vi "log analysis_gps.vi"() -> ()   [LabVIEW 2019] (continued)
31T\",12,5,5,3,04,00,20,03*fd84ab6f\n\tsystem status\tnormal 2 27.900000 0 0\trobot status\t165.672494\t122.157041\t7.863900\t0.259103\t-0.236619\t173.916290\t0.293000\t0.003000\n\t\n15:43:45.0\tlog_raw\tgps_raw\t#DUALANTENNAHEADINGA,USB3,0,47.0,FINESTEERING,2107,283443.000,02000000,d426,15824;INSUFFICIENT_OBS,NONE,-1.000000000,0.000000000,0.000000000,0.0,0.000000000,0.000000000,\"631T\",12,4,4,3,04,00,20,03*cb2f73ac\n\tsystem status\tnormal 2 27.900000 0 0\trobot status\t165.523586\t122.191427\t7.865700\t0.210877\t-0.293700\t173.825289\t0.305000\t0.013000\n\t\n15:43:45.5\tlog_raw\tgps_raw\t#DUALANTENNAHEADINGA,USB3,0,50.0,FINESTEERING,2107,283443.500,02000000,d426,15824;SOL_COMPUTED,L1_FLOAT,-1.000000000,232.711517334,45.470851898,0.0,33.751167297,39.018550873,\"631T\",12,5,5,3,04,00,20,03*51b2f499\n\tsystem status\tnormal 2 27.900000 0 0\trobot status\t165.380662\t122.222844\t7.868200\t0.351026\t-0.300668\t173.767121\t0.301000\t0.006000\n\t\n15:43:46.0\tlog_raw\tgps_raw\t#DUALANTENNAHEADINGA,USB3,0,50.0,FINESTEERING,2107,283444.000,02000000,d426,15824;INSUFFICIENT_OBS,NONE,-1.000000000,0.000000000,0.000000000,0.0,0.000000000,0.000000000,\"631T\",13,4,4,3,04,00,20,03*f1c4efa0\n\tsystem status\tnormal 2 27.900000 0 0\trobot status\t165.233504\t122.257140\t7.870500\t0.509598\t-0.309448\t173.742024\t0.303000\t0.009000\n\t\n15:43:46.5\tlog_raw\tgps_raw\t#DUALANTENNAHEADINGA,USB3,0,48.0,FINESTEERING,2107,283444.500,02000000,d426,15824;INSUFFICIENT_OBS,NONE,-1.000000000,0.000000000,0.000000000,0.0,0.000000000,0.000000000,\"631T\",13,4,4,3,04,00,20,03*63cc647c\n\tsystem status\tnormal 2 27.900000 0 0\trobot status\t165.100809\t122.287890\t7.873300\t0.523177\t-0.494729\t173.684348\t0.299000\t-0.035000\n\t\n15:43:47.0\tlog_raw\tgps_raw\t#DUALANTENNAHEADINGA,USB3,0,48.0,FINESTEERING,2107,283445.000,02000000,d426,15824;INSUFFICIENT_OBS,NONE,-1.000000000,0.000000000,0.000000000,0.0,0.000000000,0.000000000,\"631T\",13,4,4,3,04,00,20,03*d90771fc\n\tsystem status\tnormal 2 27.900000 0 0\trobot status\t164.960140\t122.320641\t7.876000\t0.439094\t-0.529708\t173.639540\t0.358000\t-0.023000\n\t\n15:43:47.5\tlog_raw\tgps_raw\t#INSPVAXA,USB3,0,43.5,FINESTEERING,2107,283445.500,02000000,471d,15824;INS_ALIGNMENT_COMPLETE,INS_RTKFIXED,37.37123259759,126.72269590770,7.8782,22.3000,0.0945,-0.3330,-0.0049,0.334033623,-0.428396374,276.205094266,0.4384,0.2941,0.5693,0.1131,0.0924,0.0780,0.0965,0.1014,4.9958,0f000001,0*eef193fc\n\tsystem status\tnormal 2 27.900000 0 0\trobot status\t164.826847\t122.347921\t7.878200\t0.334034\t-0.428396\t173.794906\t0.303000\t0.000000\n\t\n15:43:48.0\tlog_raw\tgps_raw\t#DUALANTENNAHEADINGA,USB3,0,43.5,FINESTEERING,2107,283446.000,02000000,d426,15824;INSUFFICIENT_OBS,NONE,-1.000000000,0.000000000,0.000000000,0.0,0.000000000,0.000000000,\"631T\",12,4,4,3,04,00,20,03*d5fed84d\n\tsystem status\tnormal 2 27.800000 0 0\trobot status\t164.679034\t122.378754\t7.879600\t0.256661\t-0.601518\t173.977970\t0.256000\t0.060000\n\t\n15:43:48.5\tlog_raw\tgps_raw\t#INSPVAXA,USB3,0,50.0,FINESTEERING,2107,283446.500,02000000,471d,15824;INS_ALIGNMENT_COMPLETE,INS_RTKFIXED,37.37123311226,126.72269261048,7.8801,22.3000,0.1011,-0.2963,-0.0025,0.185692893,-0.737548130,275.721839304,0.4376,0.2941,0.5694,0.1127,0.0923,0.0781,0.0965,0.1014,4.9971,0f000001,0*33922ff8\n\tsystem status\tnormal 2 27.800000 0 0\trobot status\t164.534785\t122.405047\t7.880100\t0.185693\t-0.737548\t174.278161\t0.270000\t0.050000\n\t\n15:43:49.0\tlog_raw\tgps_raw\t#DUALANTENNAHEADINGA,USB3,0,50.0,FINESTEERING,2107,283447.000,02000000,d426,15824;INSUFFICIENT_OBS,NONE,-1.000000000,0.000000000,0.000000000,0.0,0.000000000,0.000000000,\"631T\",11,4,4,3,04,00,20,03*3318e43a\n\tsystem status\tnormal 2 27.800000 0 0\trobot status\t164.391452\t122.433038\t7.880200\t0.201760\t-0.895547\t174.637577\t0.423000\t-0.172000\n\t\n15:43:49.5\tlog_raw\tgps_raw\t\tsystem status\tnormal 2 27.800000 0 0\trobot status\t164.251464\t122.459981\t7.881400\t0.307007\t-0.942643\t175.000438\t0.380000\t-0.105000\n\t\n15:43:50.0\tlog_raw\tgps_raw\t\tsystem status\tnormal 2 27.800000 0 0\trobot status\t164.109642\t122.487191\t7.882000\t0.246007\t-0.944004\t175.404925\t0.310000\t0.000000\n\t\n15:43:50.5\tlog_raw\tgps_raw\t#DUALANTENNAHEADINGA,USB3,0,51.5,FINESTEERING,2107,283448.500,02000000,d426,15824;INSUFFICIENT_OBS,NONE,-1.000000000,0.000000000,0.000000000,0.0,0.000000000,0.000000000,\"631T\",14,4,4,3,04,00,20,03*e9e47ab5\n\tsystem status\tnormal 2 27.800000 0 0\trobot status\t163.966863\t122.507000\t7.881200\t0.146187\t-0.918607\t175.866962\t0.302000\t0.000000\n\t\n15:43:51.0\tlog_raw\tgps_raw\t#DUALANTENNAHEADINGA,USB3,0,51.5,FINESTEERING,2107,283449.000,02000000,d426,15824;INSUFFICIENT_OBS,NONE,-1.000000000,0.000000000,0.000000000,0.0,0.000000000,0.000000000,\"631T\",12,4,4,3,04,00,20,03*cef36426\n\tsystem status\tnormal 2 27.800000 0 0\trobot status\t163.825609\t122.528899\t7.879700\t0.116711\t-0.792490\t176.146644\t0.187000\t0.125000\n\t\n15:43:51.5\tlog_raw\tgps_raw\t\tsystem status\tnormal 2 27.800000 0 0\trobot status\t163.693916\t122.547630\t7.877800\t0.151929\t-0.650163\t176.408867\t0.313000\t0.002000\n\t\n15:43:52.0\tlog_raw\tgps_raw\t#DUALANTENNAHEADINGA,USB3,0,49.0,FINESTEERING,2107,283450.000,02000000,d426,15824;INSUFFICIENT_OBS,NONE,-1.000000000,0.000000000,0.000000000,0.0,0.000000000,0.000000000,\"631T\",14,4,4,3,04,00,20,03*09d68f9b\n\tsystem status\tnormal 2 27.800000 0 0\trobot status\t163.555418\t122.571158\t7.876300\t0.483832\t-0.633082\t176.720348\t0.260000\t0.076000\n\t\n15:43:52.5\tlog_raw\tgps_raw\t#DUALANTENNAHEADINGA,USB3,0,49.0,FINESTEERING,2107,283450.500,02000000,d426,15824;INSUFFICIENT_OBS,NONE,-1.000000000,0.000000000,0.000000000,0.0,0.000000000,0.000000000,\"631T\",12,4,4,3,04,00,20,03*431995d1\n\tsystem status\tnormal 2 27.800000 0 0\trobot status\t163.413955\t122.592581\t7.875300\t0.523841\t-0.742821\t176.868735\t0.267000\t0.059000\n\t\n15:43:53.0\tlog_raw\tgps_raw\t#DUALANTENNAHEADINGA,USB3,0,49.0,FINESTEERING,2107,283451.000,02000000,d426,15824;INSUFFICIENT_OBS,NONE,-1.000000000,0.000000000,0.000000000,0.0,0.000000000,0.000000000,\"631T\",12,4,4,3,04,00,20,03*f9d28051\n\tsystem status\tnormal 2 27.900000 0 0\trobot status\t163.273523\t122.615568\t7.873300\t0.453873\t-0.748594\t176.979246\t0.320000\t-0.040000\n\t\n15:43:53.5\tlog_raw\tgps_raw\t#DUALANTENNAHEADINGA,USB3,0,44.5,FINESTEERING,2107,283451.500,02000000,d426,15824;INSUFFICIENT_OBS,NONE,-1.000000000,0.000000000,0.000000000,0.0,0.000000000,0.000000000,\"631T\",14,4,4,3,04,00,20,03*5c854f00\n\tsystem status\tnormal 2 27.900000 0 0\trobot status\t163.130518\t122.634911\t7.871300\t0.469672\t-0.900314\t177.008308\t0.303000\t-0.013000\n\t\n15:43:54.0\tlog_raw\tgps_raw\t#DUALANTENNAHEADINGA,USB3,0,44.5,FINESTEERING,2107,283452.000,02000000,d426,15824;INSUFFICIENT_OBS,NONE,-1.000000000,0.000000000,0.000000000,0.0,0.000000000,0.000000000,\"631T\",14,4,4,3,04,00,20,03*3dfe5332\n\tsystem status\tnormal 2 27.900000 0 0\trobot status\t162.988413\t122.656985\t7.869200\t0.628422\t-0.827167\t177.062583\t0.358000\t-0.086000\n\t\n15:43:54.5\tlog_raw\tgps_raw\t#DUALANTENNAHEADINGA,USB3,0,49.0,FINESTEERING,2107,283452.500,02000000,d426,15824;INSUFFICIENT_OBS,NONE,-1.000000000,0.000000000,0.000000000,0.0,0.000000000,0.000000000,\"631T\",12,4,4,3,04,00,20,03*98a99c63\n\tsystem status\tnormal 2 27.900000 0 0\trobot status\t162.847082\t122.675336\t7.867000\t0.701223\t-0.805865\t177.020983\t0.308000\t-0.011000\n\t\n15:43:55.0\tlog_raw\tgps_raw\t#DUALANTENNAHEADINGA,USB3,0,49.0,FINESTEERING,2107,283453.000,02000000,d426,15824;INSUFFICIENT_OBS,NONE,-1.000000000,0.000000000,0.000000000,0.0,0.000000000,0.000000000,\"631T\",10,4,4,3,04,00,20,03*56d68f12\n\tsystem status\tnormal 2 27.900000 0 0\trobot status\t162.707913\t122.695365\t7.863400\t0.653811\t-0.817944\t176.906378\t0.285000\t-0.006000\n\t\n15:43:55.5\tlog_raw\tgps_raw\t#DUALANTENNAHEADINGA,USB3,0,50.0,FINESTEERING,2107,283453.500,02000000,d426,15824;INSUFFICIENT_OBS,NONE,-1.000000000,0.000000000,0.000000000,0.0,0.000000000,0.000000000,\"631T\",9,4,4,3,04,00,20,02*71c65a10\n\tsystem status\tnormal 2 27.900000 0 0\trobot status\t162.567512\t122.713036\t7.859600\t0.640293\t-0.840166\t176.803743\t0.287000\t-0.006000\n\t\n15:43:56.0\tlog_raw\tgps_raw\t#DUALANTENNAHEADINGA,USB3,0,50.0,FINESTEERING,2107,283454.000,02000000,d426,15824;INSUFFICIENT_OBS,NONE,-1.000000000,0.000000000,0.000000000,0.0,0.000000000,0.000000000,\"631T\",10,4,4,3,04,00,20,03*adf0db7d\n\tsystem status\tnormal 2 27.900000 0 0\trobot status\t162.462286\t122.731023\t7.856300\t0.648331\t-0.862744\t176.715837\t0.257000\t0.003000\n\t\n15:43:56.5\tlog_raw\tgps_raw\t#DUALANTENNAHEADINGA,USB3,0,53.5,FINESTEERING,2107,283454.500,02000000,d426,15824;INSUFFICIENT_OBS,NONE,-1.000000000,0.000000000,0.000000000,0.0,0.000000000,0.000000000,\"631T\",10,4,4,3,04,00,20,03*83545704\n\tsystem status\tnormal 2 27.900000 0 0\trobot status\t162.317691\t122.747222\t7.853100\t0.502604\t-0.882304\t176.698904\t0.312000\t-0.030000\n\t\n15:43:57.0\tlog_raw\tgps_raw\t#DUALANTENNAHEADINGA,USB3,0,53.5,FINESTEERING,2107,283455.000,02000000,d426,15824;INSUFFICIENT_OBS,NONE,-1.000000000,0.000000000,0.000000000,0.0,0.000000000,0.000000000,\"631T\",10,4,4,3,04,00,20,03*399f4284\n\tsystem status\tnormal 2 27.900000 0 0\trobot status\t162.177621\t122.765962\t7.848800\t0.462674\t-0.849181\t176.541164\t0.296000\t-0.007000\n\t\n15:43:57.5\tlog_raw\tgps_raw\t#DUALANTENNAHEADINGA,USB3,0,53.0,FINESTEERING,2107,283455.500,02000000,d426,15824;INSUFFICIENT_OBS,NONE,-1.000000000,0.000000000,0.000000000,0.0,0.000000000,0.000000000,\"631T\",10,4,4,3,04,00,20,03*bbf6b511\n\tsystem status\tnormal 2 27.900000 0 0\trobot status\t162.042961\t122.783351\t7.845600\t0.471260\t-0.741428\t176.451320\t0.306000\t-0.003000\n\t\n15:43:58.0\tlog_raw\tgps_raw\t#DUALANTENNAHEADINGA,USB3,0,53.0,FINESTEERING,2107,283456.000,02000000,d426,15824;INSUFFICIENT_OBS,NONE,-1.000000000,0.000000000,0.000000000,0.0,0.000000000,0.000000000,\"631T\",10,4,4,3,04,00,20,03*da8da923\n\tsystem status\tnormal 2 27.900000 0 0\trobot status\t161.898614\t122.802999\t7.842000\t0.376839\t-0.675596\t176.320728\t0.295000\t-0.010000\n\t\n15:43:58.5\tlog_raw\tgps_raw\t#DUALANTENNAHEADINGA,USB3,0,50.5,FINESTEERING,2107,283456.500,02000000,d426,15824;INSUFFICIENT_OBS,NONE,-1.000000000,0.000000000,0.000000000,0.0,0.000000000,0.000000000,\"631T\",10,4,4,3,04,00,20,03*f429255a\n\tsystem status\tnormal 2 27.900000 0 0\trobot status\t161.764410\t122.820069\t7.837800\t0.218441\t-0.529178\t176.132166\t0.306000\t-0.016000\n\t\n15:43:59.0\tlog_raw\tgps_raw\t#DUALANTENNAHEADINGA,USB3,0,50.5,FINESTEERING,2107,283457.000,02000000,d426,15824;INSUFFICIENT_OBS,NONE,-1.000000000,0.000000000,0.000000000,0.0,0.000000000,0.000000000,\"631T\",11,4,4,3,04,00,20,03*9900b082\n\tsystem status\tnormal 2 27.900000 0 0\trobot status\t161.620308\t122.839916\t7.833300\t0.041782\t-0.506976\t175.942397\t0.298000\t-0.010000\n\t\n15:43:59.5\tlog_raw\tgps_raw\t#DUALANTENNAHEADINGA,USB3,0,52.0,FINESTEERING,2107,283457.500,02000000,d426,15824;INSUFFICIENT_OBS,NONE,-1.000000000,0.000000000,0.000000000,0.0,0.000000000,0.000000000,\"631T\",11,4,4,3,04,00,20,03*d3e0ea5f\n\tsystem status\tnormal 2 27.900000 0 0\trobot status\t161.478382\t122.859023\t7.830000\t0.076043\t-0.364293\t175.707938\t0.306000\t-0.023000\n\t\n15:44:00.0\tlog_raw\tgps_raw\t#DUALANTENNAHEADINGA,USB3,0,52.0,FINESTEERING,2107,283458.000,02000000,d426,15824;INSUFFICIENT_OBS,NONE,-1.000000000,0.000000000,0.000000000,0.0,0.000000000,0.000000000,\"631T\",12,4,4,3,04,00,20,02*d2f97f3d\n\tsystem status\tnormal 2 27.900000 0 0\trobot status\t161.335080\t122.881838\t7.825800\t0.229097\t-0.118774\t175.500608\t0.291000\t-0.009000\n\t\n15:44:00.5\tlog_raw\tgps_raw\t#INSPVAXA,USB3,0,50.0,FINESTEERING,2107,283458.550,02000000,471d,15824;INS_ALIGNMENT_COMPLETE,INS_RTKFIXED,37.37123761110,126.72265482999,7.8240,22.3000,0.0859,-0.2308,-0.0155,0.304728357,-0.212159203,274.715146909,0.4465,0.2951,0.5711,0.1136,0.0925,0.0781,0.0966,0.1016,5.0109,0f000001,0*14308c9c\n\tsystem status\tnormal 2 27.900000 0 0\trobot status\t161.188251\t122.904414\t7.824000\t0.304728\t-0.212159\t175.284853\t0.273000\t-0.049000\n\t\n15:44:01.0\tlog_raw\tgps_raw\t#INSPVAXA,USB3,0,50.0,FINESTEERING,2107,283459.050,02000000,471d,15824;INS_ALIGNMENT_COMPLETE,INS_RTKFIXED,37.37123780985,126.72265328103,7.8227,22.3000,0.0882,-0.3585,-0.0269,0.289946645,-0.080144409,275.013875175,0.4463,0.2950,0.5710,0.1135,0.0925,0.0781,0.0966,0.1016,5.0117,0f000001,0*9875c775\n\tsystem status\tnormal 2 27.900000 0 0\trobot status\t161.051046\t122.926475\t7.822700\t0.289947\t-0.080144\t174.986125\t0.314000\t-0.036000\n\t\n15:44:01.5\tlog_raw\tgps_raw\t#INSPVAXA,USB3,0,50.5,FINESTEERING,2107,283459.550,02000000,471d,15824;INS_ALIGNMENT_COMPLETE,INS_RTKFIXED,37.37123799841,126.72265173838,7.8223,22.3000,0.0838,-0.2861,-0.0112,0.173844892,-0.010609871,275.281152331,0.4463,0.2950,0.5710,0.1135,0.0925,0.0781,0.0966,0.1016,5.0117,0f000001,0*d5666360\n\tsystem status\tnormal 2 27.900000 0 0\trobot status\t160.914401\t122.947405\t7.822300\t0.173845\t-0.010610\t174.718848\t0.286000\t0.000000\n\t\n15:44:02.0\tlog_raw\tgps_raw\t#INSPVAXA,USB3,0,50.5,FINESTEERING,2107,283460.050,02000000,471d,15824;INS_ALIGNMENT_COMPLETE,INS_RTKFIXED,37.37123822343,126.72265007400,7.8217,22.3000,0.0923,-0.2835,-0.0262,0.253668906,0.084108634,275.465582577,0.4457,0.2949,0.5709,0.1137,0.0925,0.0781,0.0966,0.1016,5.0129,0f000001,0*4b6161dc\n\tsystem status\tnormal 2 27.900000 0 0\trobot status\t160.766973\t122.972382\t7.821700\t0.253669\t0.084109\t174.534417\t0.299000\t-0.014000\n\t\n15:44:02.5\tlog_raw\tgps_raw\t#INSPVAXA,USB3,0,51.5,FINESTEERING,2107,283460.550,02000000,471d,15824;INS_ALIGNMENT_COMPLETE,INS_RTKFIXED,37.37123844435,126.72264849525,7.8205,22.3000,0.0984,-0.3080,-0.0293,0.364026369,0.239403799,275.671224814,0.4457,0.2949,0.5709,0.1137,0.0925,0.0781,0.0966,0.1016,5.0129,0f000001,0*2bf0cdc4\n\tsystem status\tnormal 2 27.900000 0 0\trobot status\t160.627130\t122.996903\t7.820500\t0.364026\t0.239404\t174.328775\t0.309000\t0.000000\n\t\n15:44:03.0\tlog_raw\tgps_raw\t#DUALANTENNAHEADINGA,USB3,0,51.5,FINESTEERING,2107,283461.000,02000000,d426,15824;INSUFFICIENT_OBS,NONE,-1.000000000,0.000000000,0.000000000,0.0,0.000000000,0.000000000,\"631T\",13,4,4,3,04,00,20,03*e487ac9d\n\tsystem status\tnormal 2 27.900000 0 0\trobot status\t160.501038\t123.021249\t7.818200\t0.437731\t0.194917\t174.128924\t0.301000\t-0.004000\n\t\n15:44:03.5\tlog_raw\tgps_raw\t#INSPVAXA,USB3,0,47.5,FINESTEERING,2107,283461.550,02000000,471d,15824;INS_ALIGNMENT_COMPLETE,INS_RTKFIXED,37.37123893716,126.72264534248,7.8162,22.3000,0.0985,-0.2963,-0.0141,0.697862948,0.169461107,276.143360178,0.4456,0.2948,0.5708,0.1136,0.0924,0.0781,0.0966,0.1015,5.0137,0f000001,0*a30b3e45\n\tsystem status\tnormal 2 27.900000 0 0\trobot status\t160.347863\t123.051603\t7.816200\t0.697863\t0.169461\t173.856640\t0.291000\t-0.009000\n\t\n15:44:04.0\tlog_raw\tgps_raw\t\tsystem status\tnormal 2 27.900000 0 0\trobot status\t160.218128\t123.078750\t7.813500\t0.737446\t-0.108971\t173.674555\t0.288000\t-0.009000\n\t\n15:44:04.5\tlog_raw\tgps_raw\t#INSPVAXA,USB3,0,43.5,FINESTEERING,2107,283462.550,02000000,471d,15824;INS_ALIGNMENT_COMPLETE,INS_RTKFIXED,37.37123942098,126.72264211433,7.8134,22.3000,0.0929,-0.3127,-0.0203,0.398142005,-0.231454144,276.636876132,0.4454,0.2949,0.5708,0.1135,0.0925,0.0781,0.0966,0.1015,5.0146,0f000001,0*24e4ed99\n\tsystem status\tnormal 2 27.900000 0 0\trobot status\t160.061918\t123.105305\t7.813400\t0.398142\t-0.231454\t173.363124\t0.312000\t0.006000\n\t\n15:44:05.0\tlog_raw\tgps_raw\t#INSPVAXA,USB3,0,43.5,FINESTEERING,2107,283463.050,02000000,471d,15824;INS_ALIGNMENT_COMPLETE,INS_RTKFIXED,37.37123965098,126.72264063011,7.8119,22.3000,0.0776,-0.1820,-0.0220,0.127573925,-0.349335206,276.957400381,0.4448,0.2950,0.5707,0.1136,0.0925,0.0781,0.0966,0.1015,5.0158,0f000001,0*86cff0c5\n\tsystem status\tnormal 2 27.900000 0 0\trobot status\t159.930449\t123.130834\t7.811900\t0.127574\t-0.349335\t173.042600\t0.092000\t-0.010000\n\t\n15:44:05.5\tlog_raw\tgps_raw\t#INSPVAXA,USB3,0,50.0,FINESTEERING,2107,283463.550,02000000,471d,15824;INS_ALIGNMENT_COMPLETE,INS_RTKFIXED,37.37123983702,126.72263968205,7.8117,22.3000,0.1160,-0.4339,-0.0234,0.042320213,-0.166110227,277.135399170,0.4448,0.2950,0.5707,0.1136,0.0925,0.0781,0.0966,0.1015,5.0158,0f000001,0*a9cde56f\n\tsystem status\tnormal 2 27.800000 0 0\trobot status\t159.846471\t123.151483\t7.811700\t0.042320\t-0.166110\t172.864601\t0.351000\t-0.033000\n\t\n15:44:06.0\tlog_raw\tgps_raw\t\tsystem status\tnormal 2 27.900000 0 0\trobot status\t159.693074\t123.182111\t7.811200\t0.143061\t-0.087094\t172.749204\t0.267000\t-0.023000\n\t\n15:44:06.5\tlog_raw\tgps_raw\t#INSPVAXA,USB3,0,50.5,FINESTEERING,2107,283464.550,02000000,471d,15824;INS_ALIGNMENT_COMPLETE,INS_RTKFIXED,37.37124035890,126.72263654398,7.8101,22.3000,0.0978,-0.3247,-0.0269,0.153067823,0.062690713,277.456657188,0.4447,0.2949,0.5707,0.1135,0.0925,0.0781,0.0966,0.1015,5.0168,0f000001,0*e25a65bd\n\tsystem status\tnormal 2 27.900000 0 0\trobot status\t159.568506\t123.209409\t7.810100\t0.153068\t0.062691\t172.543343\t0.311000\t-0.003000\n\t\n15:44:07.0\tlog_raw\tgps_raw\t\tsystem status\tnormal 2 27.900000 0 0\trobot status\t159.436087\t123.236671\t7.809800\t-0.028782\t-0.085337\t172.438609\t0.291000\t0.009000\n\t\n15:44:07.5\tlog_raw\tgps_raw\t#INSPVAXA,USB3,0,47.5,FINESTEERING,2107,283465.550,02008000,471d,15824;INS_ALIGNMENT_COMPLETE,INS_RTKFIXED,37.37124087816,126.72263323359,7.8095,22.3000,0.1048,-0.3207,-0.0188,-0.139743326,-0.216469066,277.649451326,0.4444,0.2948,0.5707,0.1135,0.0925,0.0781,0.0966,0.1015,5.0179,0f000001,0*3b3a13db\n\tsystem status\tnormal 2 27.900000 0 0\trobot status\t159.275277\t123.267045\t7.809500\t-0.139743\t-0.216469\t172.350549\t0.307000\t0.009000\n\t\n15:44:08.0\tlog_raw\tgps_raw\t#INSPVAXA,USB3,0,47.0,FINESTEERING,2107,283466.050,02008000,471d,15824;INS_ALIGNMENT_COMPLETE,INS_RTKFIXED,37.37124115647,126.72263161557,7.8102,22.3000,0.1038,-0.3165,-0.0156,-0.037052070,-0.429278496,277.644852410,0.4437,0.2948,0.5706,0.1136,0.0925,0.0781,0.0966,0.1015,5.0190,0f000001,0*71415a25\n\tsystem status\tnormal 2 27.900000 0 0\trobot status\t159.131955\t123.297935\t7.810200\t-0.037052\t-0.429278\t172.355148\t0.300000\t0.012000\n\t\n15:44:08.5\tlog_raw\tgps_raw\t\tsystem status\tnormal 2 27.900000 0 0\trobot status\t158.997671\t123.327969\t7.810800\t0.156637\t-0.605991\t172.264093\t0.301000\t0.006000\n\t\n15:44:09.0\tlog_raw\tgps_raw\t#INSPVAXA,USB3,0,46.5,FINESTEERING,2107,283467.050,02008000,471d,15824;INS_ALIGNMENT_COMPLETE,INS_RTKFIXED,37.37124175185,126.72262828673,7.8114,22.3000,0.1144,-0.3107,-0.0235,0.189502130,-0.846127382,277.724037257,0.4428,0.2947,0.5707,0.1137,0.0925,0.0781,0.0965,0.1015,5.0203,0f000001,0*123a4309\n\tsystem status\tnormal 2 27.900000 0 0\trobot status\t158.837092\t123.364019\t7.811400\t0.189502\t-0.846127\t172.275963\t0.354000\t-0.070000\n\t\n15:44:09.5\tlog_raw\tgps_raw\t#INSPVAXA,USB3,0,46.5,FINESTEERING,2107,283467.550,02008000,471d,15824;INS_ALIGNMENT_COMPLETE,INS_RTKFIXED,37.37124201534,126.72262669568,7.8140,22.3000,0.1123,-0.3073,-0.0295,0.009270111,-0.651900427,277.586297393,0.4428,0.2947,0.5707,0.1137,0.0925,0.0781,0.0965,0.1015,5.0203,0f000001,0*fbe18a0e\n\tsystem status\tnormal 2 27.800000 0 0\trobot status\t158.696160\t123.393265\t7.814000\t0.009270\t-0.651900\t172.413703\t0.400000\t-0.141000\n\t\n15:44:10.0\tlog_raw\tgps_raw\t#INSPVAXA,USB3,0,46.5,FINESTEERING,2107,283468.050,02008000,471d,15824;INS_ALIGNMENT_COMPLETE,INS_RTKFIXED,37.37124222504,126.72262566051,7.8172,22.3000,0.1108,-0.3362,-0.0087,-0.107061693,-0.300479495,277.280043662,0.4419,0.2947,0.5706,0.1134,0.0926,0.0781,0.0965,0.1015,5.0216,0f000001,0*e4f8bd3b\n\tsystem status\tnormal 2 27.700000 0 0\trobot status\t158.604466\t123.416540\t7.817200\t-0.107062\t-0.300479\t172.719956\t0.158000\t0.015000\n\t\n15:44:10.5\tlog_raw\tgps_raw\t#INSPVAXA,USB3,0,46.5,FINESTEERING,2107,283468.550,02008000,471d,15824;INS_ALIGNMENT_COMPLETE,INS_RTKFIXED,37.37124250886,126.72262396333,7.8186,22.3000,0.0904,-0.2606,-0.0155,0.241398611,-0.239914354,276.982575871,0.4419,0.2947,0.5706,0.1134,0.0926,0.0781,0.0965,0.1015,5.0216,0f000001,0*b84fac19\n\tsystem status\tnormal 2 27.800000 0 0\trobot status\t158.454133\t123.448043\t7.818600\t0.241399\t-0.239914\t173.017424\t0.291000\t-0.029000\n\t\n15:44:11.0\tlog_raw\tgps_raw\t#INSPVAXA,USB3,0,46.5,FINESTEERING,2107,283469.050,02008000,471d,15824;INS_ALIGNMENT_COMPLETE,INS_RTKFIXED,37.37124277441,126.72262234556,7.8204,22.3000,0.0912,-0.2797,-0.0071,0.371726808,-0.134537847,276.502900110,0.4420,0.2946,0.5707,0.1134,0.0925,0.0781,0.0965,0.1015,5.0228,0f000001,0*e3b85341\n\tsystem status\tnormal 2 27.800000 0 0\trobot status\t158.310833\t123.477517\t7.820400\t0.371727\t-0.134538\t173.497100\t0.328000\t-0.048000\n\t\n15:44:11.5\tlog_raw\tgps_raw\t#INSPVAXA,USB3,0,46.5,FINESTEERING,2107,283469.550,02000000,471d,15824;INS_ALIGNMENT_COMPLETE,INS_RTKFIXED,37.37124299469,126.72262074731,7.8238,22.3000,0.0920,-0.2961,-0.0076,0.268432446,-0.051624377,275.936964776,0.4420,0.2946,0.5707,0.1134,0.0925,0.0781,0.0965,0.1015,5.0228,0f000001,0*2bf39c83\n\tsystem status\tnormal 2 27.700000 0 0\trobot status\t158.169263\t123.501968\t7.823800\t0.268432\t-0.051624\t174.063035\t0.172000\t0.204000\n\t\n15:44:12.0\tlog_raw\tgps_raw\t#INSPVAXA,USB3,0,46.5,FINESTEERING,2107,283470.050,02000000,471d,15824;INS_ALIGNMENT_COMPLETE,INS_RTKFIXED,37.37124320185,126.72261913294,7.8277,22.3000,0.1016,-0.3039,-0.0081,0.097334282,-0.040914824,275.470071577,0.4421,0.2945,0.5705,0.1133,0.0925,0.0781,0.0965,0.1015,5.0240,0f000001,0*fba59bc0\n\tsystem status\tnormal 2 27.700000 0 0\trobot status\t158.026264\t123.524962\t7.827700\t0.097334\t-0.040915\t174.529928\t0.396000\t-0.142000\n\t\n15:44:12.5\tlog_raw\tgps_raw\t#INSPVAXA,USB3,0,46.0,FINESTEERING,2107,283470.550,02000000,471d,15824;INS_ALIGNMENT_COMPLETE,INS_RTKFIXED,37.37124338791,126.72261753041,7.8308,22.3000,0.0952,-0.3085,-0.0166,0.133198761,-0.149300004,274.919636182,0.4421,0.2945,0.5705,0.1133,0.0925,0.0781,0.0965,0.1015,5.0240,0f000001,0*42261ade\n\tsystem status\tnormal 2 27.700000 0 0\trobot status\t157.884315\t123.545615\t7.830800\t0.133199\t-0.149300\t175.080364\t0.328000\t-0.031000\n\t\n15:44:13.0\tlog_raw\tgps_raw\t#INSPVAXA,USB3,0,46.0,FINESTEERING,2107,283471.050,02000000,471d,15824;INS_ALIGNMENT_COMPLETE,INS_RTKFIXED,37.37124356076,126.72261595668,7.8336,22.3000,0.0792,-0.2815,-0.0153,0.105112248,-0.115677362,274.303120166,0.4420,0.2946,0.5706,0.1132,0.0925,0.0781,0.0964,0.1015,5.0248,0f000001,0*c06838c2\n\tsystem status\tnormal 2 27.700000 0 0\trobot status\t157.744917\t123.564801\t7.833600\t0.105112\t-0.115677\t175.696880\t0.269000\t0.042000\n\t\n15:44:13.5\tlog_raw\tgps_raw\t#INSPVAXA,USB3,0,48.0,FINESTEERING,2107,283471.550,02000000,471d,15824;INS_ALIGNMENT_COMPLETE,INS_RTKFIXED,37.37124371844,126.72261435668,7.8362,22.3000,0.0861,-0.3146,0.0012,0.009847777,-0.154362350,273.837649570,0.4420,0.2946,0.5706,0.1132,0.0925,0.0781,0.0964,0.1015,5.0248,0f000001,0*248758d2\n\tsystem status\tnormal 2 27.800000 0 0\trobot status\t157.603191\t123.582304\t7.836200\t0.009848\t-0.154362\t176.162350\t0.254000\t0.082000\n\t\n15:44:14.0\tlog_raw\tgps_raw\t#INSPVAXA,USB3,0,48.0,FINESTEERING,2107,283472.050,02000000,471d,15824;INS_ALIGNMENT_COMPLETE,INS_RTKFIXED,37.37124388873,126.72261272959,7.8390,22.3000,0.0744,-0.3068,0.0071,0.047718600,-0.362449077,273.522239359,0.4416,0.2945,0.5705,0.1131,0.0924,0.0781,0.0964,0.1014,5.0253,0f000001,0*b034cfcb\n\tsystem status\tnormal 2 27.800000 0 0\trobot status\t157.459066\t123.601206\t7.839000\t0.047719\t-0.362449\t176.477761\t0.261000\t0.067000\n\t\n15:44:14.5\tlog_raw\tgps_raw\t\tsystem status\tnormal 2 27.900000 0 0\trobot status\t157.351393\t123.616406\t7.841000\t0.156868\t-0.620801\t176.811707\t0.118000\t0.023000\n\t\n15:44:15.0\tlog_raw\tgps_raw\t#INSPVAXA,USB3,0,48.5,FINESTEERING,2107,283473.050,02000000,471d,15824;INS_ALIGNMENT_COMPLETE,INS_RTKFIXED,37.37124418423,126.72260986099,7.8423,22.3000,0.0465,-0.2147,-0.0152,-0.064754413,-0.661648789,273.035495694,0.4408,0.2944,0.5705,0.1130,0.0925,0.0781,0.0964,0.1014,5.0261,0f000001,0*8452aba9\n\tsystem status\tnormal 2 27.800000 0 0\trobot status\t157.204970\t123.634007\t7.842300\t-0.064754\t-0.661649\t176.964504\t0.310000\t-0.063000\n\t\n15:44:15.5\tlog_raw\tgps_raw\t#INSPVAXA,USB3,0,49.5,FINESTEERING,2107,283473.550,02000000,471d,15824;INS_ALIGNMENT_COMPLETE,INS_RTKFIXED,37.37124432645,126.72260825595,7.8450,22.3000,0.0577,-0.2717,-0.0116,-0.371304457,-0.586321968,273.022512586,0.4408,0.2944,0.5705,0.1130,0.0925,0.0781,0.0964,0.1014,5.0261,0f000001,0*dc18a2a0\n\tsystem status\tnormal 2 27.900000 0 0\trobot status\t157.062799\t123.649793\t7.845000\t-0.371304\t-0.586322\t176.977487\t0.282000\t0.058000\n\t\n15:44:16.0\tlog_raw\tgps_raw\t#INSPVAXA,USB3,0,49.5,FINESTEERING,2107,283474.050,02000000,471d,15824;INS_ALIGNMENT_COMPLETE,INS_RTKFIXED,37.37124450056,126.72260664706,7.8482,22.3000,0.0746,-0.3111,-0.0073,-0.324886266,-0.572903828,273.001550597,0.4404,0.2944,0.5705,0.1132,0.0924,0.0781,0.0964,0.1014,5.0269,0f000001,0*6a9d6035\n\tsystem status\tnormal 2 27.900000 0 0\trobot status\t156.920286\t123.669120\t7.848200\t-0.324886\t-0.572904\t176.998449\t0.371000\t-0.100000\n\t\n15:44:16.5\tlog_raw\tgps_raw\t#INSPVAXA,USB3,0,47.5,FINESTEERING,2107,283474.550,02000000,471d,15824;INS_ALIGNMENT_COMPLETE,INS_RTKFIXED,37.37124465803,126.72260513334,7.8520,22.3000,0.0754,-0.3176,-0.0107,-0.183521843,-0.419147720,273.001614908,0.4404,0.2944,0.5705,0.1132,0.0924,0.0781,0.0964,0.1014,5.0269,0f000001,0*c3ef68c2\n\tsystem status\tnormal 2 27.900000 0 0\trobot status\t156.786203\t123.686599\t7.852000\t-0.183522\t-0.419148\t176.998385\t0.303000\t0.000000\n\t\n15:44:17.0\tlog_raw\tgps_raw\t#INSPVAXA,USB3,0,47.5,FINESTEERING,2107,283475.050,02000000,471d,15824;INS_ALIGNMENT_COMPLETE,INS_RTKFIXED,37.37124482420,126.72260357530,7.8549,22.3000,0.0753,-0.2803,-0.0146,-0.241068696,-0.296923689,273.106112886,0.4399,0.2945,0.5706,0.1130,0.0924,0.0781,0.0964,0.1014,5.0279,0f000001,0*9f37bee3\n\tsystem status\tnormal 2 27.900000 0 0\trobot status\t156.648194\t123.705044\t7.854900\t-0.241069\t-0.296924\t176.893887\t0.277000\t0.000000\n\t\n15:44:17.5\tlog_raw\tgps_raw\t#INSPVAXA,USB3,0,47.5,FINESTEERING,2107,283475.550,02000000,471d,15824;INS_ALIGNMENT_COMPLETE,INS_RTKFIXED,37.37124499067,126.72260199547,7.8565,22.3000,0.0685,-0.2996,-0.0135,-0.434680931,-0.247748012,273.252507934,0.4399,0.2945,0.5706,0.1130,0.0924,0.0781,0.0964,0.1014,5.0279,0f000001,0*f6dcb523\n\tsystem status\tnormal 2 27.900000 0 0\trobot status\t156.508255\t123.723522\t7.856500\t-0.434681\t-0.247748\t176.747492\t0.297000\t-0.008000\n\t\n15:44:18.0\tlog_raw\tgps_raw\t#INSPVAXA,USB3,0,47.5,FINESTEERING,2107,283476.050,02000000,471d,15824;INS_ALIGNMENT_COMPLETE,INS_RTKFIXED,37.37124517702,126.72260043999,7.8594,22.3000,0.0731,-0.2995,-0.0095,-0.441036624,-0.242977977,273.321134070,0.4399,0.2945,0.5707,0.1130,0.0924,0.0781,0.0964,0.1014,5.0290,0f000001,0*df4d40ec\n\tsystem status\tnormal 2 27.900000 0 0\trobot status\t156.370474\t123.744207\t7.859400\t-0.441037\t-0.242978\t176.678866\t0.296000\t-0.012000\n\t\n15:44:18.5\tlog_raw\tgps_raw\t#INSPVAXA,USB3,0,50.0,FINESTEERING,2107,283476.550,02000000,471d,15824;INS_ALIGNMENT_COMPLETE,INS_RTKFIXED,37.37124535364,126.72259887050,7.8616,22.3000,0.0731,-0.2996,-0.0100,-0.412710306,-0.285107992,273.399842482,0.4399,0.2945,0.5707,0.1130,0.0924,0.0781,0.0964,0.1014,5.0290,0f000001,0*4ef28dbb\n\tsystem status\tnormal 2 27.900000 0 0\trobot status\t156.231451\t123.763811\t7.861600\t-0.412710\t-0.285108\t176.600158\t0.296000\t-0.011000\n\t\n15:44:19.0\tlog_raw\tgps_raw\t\tsystem status\tnormal 2 27.900000 0 0\trobot status\t156.092059\t123.783361\t7.862700\t-0.521984\t-0.483265\t176.481711\t0.297000\t-0.011000\n\t\n15:44:19.5\tlog_raw\tgps_raw\t#INSPVAXA,USB3,0,51.0,FINESTEERING,2107,283477.550,02000000,471d,15824;INS_ALIGNMENT_COMPLETE,INS_RTKFIXED,37.37124569782,126.72259576074,7.8655,22.3000,0.0695,-0.3003,-0.0075,-0.469235251,-0.455743841,273.579264680,0.4397,0.2945,0.5707,0.1130,0.0924,0.0781,0.0964,0.1014,5.0303,0f000001,0*db0f6a2f\n\tsystem status\tnormal 2 27.900000 0 0\trobot status\t155.955993\t123.802015\t7.865500\t-0.469235\t-0.455744\t176.420735\t0.300000\t0.000000\n\t\n15:44:20.0\tlog_raw\tgps_raw\t#INSPVAXA,USB3,0,51.0,FINESTEERING,2107,283478.050,02000000,471d,15824;INS_ALIGNMENT_COMPLETE,INS_RTKFIXED,37.37124587328,126.72259421546,7.8690,22.3000,0.0786,-0.2811,0.0029,-0.458800403,-0.268524381,273.658587255,0.4407,0.2947,0.5709,0.1132,0.0924,0.0781,0.0964,0.1014,5.0316,0f000001,0*f403e502\n\tsystem status\tnormal 2 27.900000 0 0\trobot status\t155.819115\t123.821491\t7.869000\t-0.458800\t-0.268524\t176.341413\t0.293000\t-0.010000\n\t\n15:44:20.5\tlog_raw\tgps_raw\t#INSPVAXA,USB3,0,51.0,FINESTEERING,2107,283478.550,02000000,471d,15824;INS_ALIGNMENT_COMPLETE,INS_RTKFIXED,37.37124604525,126.72259266223,7.8723,22.3000,0.0753,-0.2945,0.0030,-0.462352826,-0.136958884,273.744107735,0.4407,0.2947,0.5709,0.1132,0.0924,0.0781,0.0964,0.1014,5.0316,0f000001,0*3bf5fab5\n\tsystem status\tnormal 2 27.900000 0 0\trobot status\t155.681532\t123.840580\t7.872300\t-0.462353\t-0.136959\t176.255892\t0.301000\t-0.002000\n\t\n15:44:21.0\tlog_raw\tgps_raw\t#INSPVAXA,USB3,0,51.0,FINESTEERING,2107,283479.050,02000000,471d,15824;INS_ALIGNMENT_COMPLETE,INS_RTKFIXED,37.37124622444,126.72259108516,7.8745,22.3000,0.0782,-0.2955,0.0000,-0.529822830,0.178727443,273.870016111,0.4415,0.2947,0.5709,0.1133,0.0924,0.0781,0.0964,0.1014,5.0329,0f000001,0*0db861ca\n\tsystem status\tnormal 2 27.900000 0 0\trobot status\t155.541838\t123.860470\t7.874500\t-0.529823\t0.178727\t176.129984\t0.298000\t-0.003000\n\t\n15:44:21.5\tlog_raw\tgps_raw\t#INSPVAXA,USB3,0,51.0,FINESTEERING,2107,283479.550,02000000,471d,15824;INS_ALIGNMENT_COMPLETE,INS_RTKFIXED,37.37124640170,126.72258950006,7.8775,22.3000,0.0805,-0.3037,0.0007,-0.509921072,0.195230583,273.949901234,0.4415,0.2947,0.5709,0.1133,0.0924,0.0781,0.0964,0.1014,5.0329,0f000001,0*077866b6\n\tsystem status\tnormal 2 27.900000 0 0\trobot status\t155.401433\t123.880145\t7.877500\t-0.509921\t0.195231\t176.050099\t0.297000\t-0.005000\n\t\n15:44:22.0\tlog_raw\tgps_raw\t#INSPVAXA,USB3,0,51.0,FINESTEERING,2107,283480.050,02000000,471d,15824;INS_ALIGNMENT_COMPLETE,INS_RTKFIXED,37.37124659299,126.72258788570,7.8812,22.3000,0.0832,-0.3022,-0.0023,-0.414591825,-0.152431490,274.036956074,0.4426,0.2949,0.5711,0.1133,0.0924,0.0781,0.0964,0.1014,5.0343,0f000001,0*6e70f737\n\tsystem status\tnormal 2 27.900000 0 0\trobot status\t155.258435\t123.901378\t7.881200\t-0.414592\t-0.152431\t175.963044\t0.297000\t-0.005000\n\t\n15:44:22.5\tlog_raw\tgps_raw\t\tsystem status\tnormal 2 27.900000 0 0\trobot status\t155.115460\t123.922017\t7.885700\t-0.361174\t-0.341781\t175.867746\t0.294000\t-0.007000\n\t\n15:44:23.0\tlog_raw\tgps_raw\t\tsystem status\tnormal 2 27.900000 0 0\trobot status\t154.969729\t123.942945\t7.890800\t-0.432586\t-0.470805\t175.774628\t0.299000\t-0.001000\n\t\n15:44:23.5\tlog_raw\tgps_raw\t#INSPVAXA,USB3,0,50.0,FINESTEERING,2107,283481.550,02000000,471d,15824;INS_ALIGNMENT_COMPLETE,INS_RTKFIXED,37.37124714529,126.72258299767,7.8939,22.3000,0.0873,-0.3069,-0.0133,-0.586135229,-0.604059291,274.319909589,0.4441,0.2951,0.5712,0.1135,0.0925,0.0781,0.0964,0.1015,5.0357,0f000001,0*8645286f\n\tsystem status\tnormal 2 27.900000 0 0\trobot status\t154.825461\t123.962683\t7.893900\t-0.586135\t-0.604059\t175.680090\t0.298000\t0.000000\n\t\n15:44:24.0\tlog_raw\tgps_raw\t\tsystem status\tnormal 2 27.900000 0 0\trobot status\t154.706863\t123.982418\t7.896300\t-0.558753\t-0.549010\t175.623992\t0.270000\t0.035000\n\t\n15:44:24.5\tlog_raw\tgps_raw\t#INSPVAXA,USB3,0,51.0,FINESTEERING,2107,283482.550,02000000,471d,15824;INS_ALIGNMENT_COMPLETE,INS_RTKFIXED,37.37124752948,126.72258005871,7.9006,22.3000,0.0687,-0.3152,0.0109,-0.135978920,-0.255823048,274.401094363,0.4449,0.2953,0.5713,0.1139,0.0925,0.0782,0.0964,0.1015,5.0373,0f000001,0*5cec8015\n\tsystem status\tnormal 2 27.900000 0 0\trobot status\t154.565133\t124.005327\t7.900600\t-0.135979\t-0.255823\t175.598906\t0.317000\t-0.006000\n\t\n15:44:25.0\tlog_raw\tgps_raw\t\tsystem status\tnormal 2 27.900000 0 0\trobot status\t154.432681\t124.026328\t7.906400\t-0.058621\t-0.060747\t175.655941\t0.308000\t0.012000\n\t\n15:44:25.5\tlog_raw\tgps_raw\t\tsystem status\tnormal 2 27.900000 0 0\trobot status\t154.287763\t124.047374\t7.911400\t-0.201590\t0.007494\t175.603374\t0.296000\t0.001000\n\t\n15:44:26.0\tlog_raw\tgps_raw\t#INSPVAXA,USB3,0,51.5,FINESTEERING,2107,283484.050,02000000,471d,15824;INS_ALIGNMENT_COMPLETE,INS_RTKFIXED,37.37124809880,126.72257534904,7.9142,22.3000,0.0705,-0.2771,0.0043,-0.387988149,0.243310051,274.386615848,0.4464,0.2955,0.5716,0.1138,0.0925,0.0782,0.0964,0.1015,5.0399,0f000001,0*6b4a4f7e\n\tsystem status\tnormal 2 27.900000 0 0\trobot status\t154.147958\t124.068521\t7.914200\t-0.387988\t0.243310\t175.613384\t0.283000\t0.023000\n\t\n15:44:26.5\tlog_raw\tgps_raw\t\tsystem status\tnormal 2 27.900000 0 0\trobot status\t154.008427\t124.090632\t7.917600\t-0.234821\t0.492649\t175.741644\t0.260000\t0.066000\n\t\n15:44:27.0\tlog_raw\tgps_raw\t#INSPVAXA,USB3,0,53.5,FINESTEERING,2107,283485.050,02000000,471d,15824;INS_ALIGNMENT_COMPLETE,INS_RTKFIXED,37.37124849221,126.72257218238,7.9219,22.3000,0.0806,-0.2954,-0.0022,-0.251628518,0.390951997,274.060594650,0.4471,0.2956,0.5717,0.1137,0.0925,0.0782,0.0964,0.1014,5.0410,0f000001,0*78d5c28f\n\tsystem status\tnormal 2 27.800000 0 0\trobot status\t153.867461\t124.112188\t7.921900\t-0.251629\t0.390952\t175.939405\t0.285000\t0.033000\n\t\n15:44:27.5\tlog_raw\tgps_raw\t#INSPVAXA,USB3,0,51.0,FINESTEERING,2107,283485.550,02000000,471d,15824;INS_ALIGNMENT_COMPLETE,INS_RTKFIXED,37.37124867338,126.72257057546,7.9253,22.3000,0.0807,-0.2982,0.0046,-0.297126660,0.143555432,273.789468415,0.4471,0.2956,0.5717,0.1137,0.0925,0.0782,0.0964,0.1014,5.0410,0f000001,0*c848650b\n\tsystem status\tnormal 2 27.800000 0 0\trobot status\t153.725122\t124.132298\t7.925300\t-0.297127\t0.143555\t176.210532\t0.284000\t0.041000\n\t\n15:44:28.0\tlog_raw\tgps_raw\t#INSPVAXA,USB3,0,46.0,FINESTEERING,2107,283486.050,02000000,471d,15824;INS_ALIGNMENT_COMPLETE,INS_RTKFIXED,37.37124886174,126.72256897160,7.9281,22.3000,0.0774,-0.2942,-0.0013,-0.283569757,0.106976902,273.570280777,0.4473,0.2956,0.5718,0.1136,0.0925,0.0782,0.0964,0.1014,5.0421,0f000001,0*a5ad5170\n\tsystem status\tnormal 2 27.800000 0 0\trobot status\t153.583055\t124.153206\t7.928100\t-0.283570\t0.106977\t176.429719\t0.284000\t0.024000\n\t\n15:44:28.5\tlog_raw\tgps_raw\t\tsystem status\tnormal 2 27.800000 0 0\trobot status\t153.456036\t124.172210\t7.932700\t-0.181705\t-0.025951\t176.745654\t0.218000\t-0.018000\n\t\n15:44:29.0\tlog_raw\tgps_raw\t\tsystem status\tnormal 2 27.800000 0 0\trobot status\t153.313952\t124.191036\t7.937500\t-0.275667\t-0.175412\t177.043665\t0.353000\t-0.119000\n\t\n15:44:29.5\tlog_raw\tgps_raw\t#INSPVAXA,USB3,0,48.0,FINESTEERING,2107,283487.550,02000000,471d,15824;INS_ALIGNMENT_COMPLETE,INS_RTKFIXED,37.37124935038,126.72256433363,7.9396,22.3000,0.0684,-0.2764,-0.0073,-0.272700392,-0.138830686,272.596264652,0.4472,0.2956,0.5720,0.1137,0.0925,0.0782,0.0964,0.1014,5.0432,0f000001,0*7a2c3ea8\n\tsystem status\tnormal 2 27.800000 0 0\trobot status\t153.172231\t124.207445\t7.939600\t-0.272700\t-0.138831\t177.403735\t0.241000\t0.087000\n\t\n15:44:30.0\tlog_raw\tgps_raw\t#INSPVAXA,USB3,0,48.0,FINESTEERING,2107,283488.050,02000000,471d,15824;INS_ALIGNMENT_COMPLETE,INS_RTKFIXED,37.37124950186,126.72256271851,7.9401,22.3000,0.0702,-0.2701,-0.0123,-0.306984619,-0.156481327,272.240352171,0.4472,0.2957,0.5722,0.1136,0.0925,0.0782,0.0964,0.1014,5.0443,0f000001,0*50a165ff\n\tsystem status\tnormal 2 27.800000 0 0\trobot status\t153.029167\t124.224259\t7.940100\t-0.306985\t-0.156481\t177.759648\t0.216000\t0.122000\n\t\n15:44:30.5\tlog_raw\tgps_raw\t#INSPVAXA,USB3,0,48.5,FINESTEERING,2107,283488.550,02000000,471d,15824;INS_ALIGNMENT_COMPLETE,INS_RTKFIXED,37.37124963696,126.72256112600,7.9399,22.3000,0.0634,-0.2924,-0.0061,-0.348692985,-0.211479337,271.855613875,0.4472,0.2957,0.5722,0.1136,0.0925,0.0782,0.0964,0.1014,5.0443,0f000001,0*ed71010c\n\tsystem status\tnormal 2 27.800000 0 0\trobot status\t152.888105\t124.239256\t7.939900\t-0.348693\t-0.211479\t178.144386\t0.325000\t-0.032000\n\t\n15:44:31.0\tlog_raw\tgps_raw\t\tsystem status\tnormal 2 27.800000 0 0\trobot status\t152.744662\t124.255774\t7.940000\t-0.314606\t-0.444516\t178.512358\t0.280000\t0.041000\n\t\n15:44:31.5\tlog_raw\tgps_raw\t#INSPVAXA,USB3,0,49.0,FINESTEERING,2107,283489.550,02000000,471d,15824;INS_ALIGNMENT_COMPLETE,INS_RTKFIXED,37.37124992844,126.72255789438,7.9412,22.3000,0.0625,-0.2932,0.0092,-0.217423535,-0.472312164,271.147208708,0.4467,0.2958,0.5722,0.1138,0.0925,0.0782,0.0964,0.1014,5.0457,0f000001,0*6d85d9a8\n\tsystem status\tnormal 2 27.800000 0 0\trobot status\t152.601853\t124.271611\t7.941200\t-0.217424\t-0.472312\t178.852791\t0.279000\t0.045000\n\t\n15:44:32.0\tlog_raw\tgps_raw\t#INSPVAXA,USB3,0,49.0,FINESTEERING,2107,283490.050,02000000,471d,15824;INS_ALIGNMENT_COMPLETE,INS_RTKFIXED,37.37125008339,126.72255625341,7.9419,22.3000,0.0636,-0.2955,0.0152,0.008734422,-0.613623948,270.920387351,0.4456,0.2958,0.5721,0.1138,0.0926,0.0782,0.0964,0.1014,5.0473,0f000001,0*aa76f15f\n\tsystem status\tnormal 2 27.800000 0 0\trobot status\t152.456499\t124.288811\t7.941900\t0.008734\t-0.613624\t179.079613\t0.211000\t0.138000\n\t\n15:44:32.5\tlog_raw\tgps_raw\t#INSPVAXA,USB3,0,52.5,FINESTEERING,2107,283490.550,02000000,471d,15824;INS_ALIGNMENT_COMPLETE,INS_RTKFIXED,37.37125019673,126.72255461280,7.9407,22.3000,0.0735,-0.3073,0.0114,-0.028034352,-0.928675652,270.685326293,0.4456,0.2958,0.5721,0.1138,0.0926,0.0782,0.0964,0.1014,5.0473,0f000001,0*cd41eb0e\n\tsystem status\tnormal 2 27.800000 0 0\trobot status\t152.311176\t124.301392\t7.940700\t-0.028034\t-0.928676\t179.314674\t0.376000\t-0.112000\n\t\n15:44:33.0\tlog_raw\tgps_raw\t\tsystem status\tnormal 2 27.800000 0 0\trobot status\t152.168909\t124.314808\t7.939900\t0.041397\t-0.895426\t179.513290\t0.212000\t0.080000\n\t\n15:44:33.5\tlog_raw\tgps_raw\t\tsystem status\tnormal 2 27.800000 0 0\trobot status\t152.056783\t124.324914\t7.939800\t0.007412\t-0.701328\t179.619806\t0.346000\t0.046000\n\t\n15:44:34.0\tlog_raw\tgps_raw\t\tsystem status\tnormal 2 27.800000 0 0\trobot status\t151.913452\t124.336030\t7.939500\t-0.070577\t-0.865666\t179.882663\t0.321000\t0.017000\n\t\n15:44:34.5\tlog_raw\tgps_raw\t\tsystem status\tnormal 2 27.800000 0 0\trobot status\t151.769263\t124.347275\t7.937600\t0.102153\t-0.775155\t-179.880488\t0.301000\t0.027000\n\t\n15:44:35.0\tlog_raw\tgps_raw\t\tsystem status\tnormal 2 27.800000 0 0\trobot status\t151.624728\t124.360279\t7.935600\t0.349982\t-0.456188\t-179.781906\t0.290000\t0.011000\n\t\n15:44:35.5\tlog_raw\tgps_raw\t\tsystem status\tnormal 2 27.900000 0 0\trobot status\t151.477074\t124.372326\t7.935400\t0.473171\t-0.513284\t-179.708584\t0.253000\t0.057000\n\t\n15:44:36.0\tlog_raw\tgps_raw\t\tsystem status\tnormal 2 27.900000 0 0\trobot status\t151.330172\t124.383551\t7.935300\t0.222440\t-0.540631\t-179.688750\t0.216000\t0.121000\n\t\n15:44:36.5\tlog_raw\tgps_raw\t\tsystem status\tnormal 2 27.900000 0 0\trobot status\t151.185645\t124.394282\t7.934100\t0.014517\t-0.469071\t-179.638862\t0.249000\t0.072000\n\t\n15:44:37.0\tlog_raw\tgps_raw\t\tsystem status\tnormal 2 27.900000 0 0\trobot status\t151.037302\t124.407488\t7.933000\t-0.004087\t-0.425392\t-179.646446\t0.365000\t-0.106000\n\t\n15:44:37.5\tlog_raw\tgps_raw\t\tsystem status\tnormal 2 27.900000 0 0\trobot status\t150.891323\t124.419002\t7.930600\t-0.059967\t-0.511341\t-179.609054\t0.284000\t0.014000\n\t\n15:44:38.0\tlog_raw\tgps_raw\t\tsystem status\tnormal 2 27.800000 0 0\trobot status\t150.782346\t124.431492\t7.929000\t-0.127004\t-0.444900\t-179.444381\t0.303000\t0.003000\n
